vi "RichToFlatnise_StatusInfo.vi"(5 "OutputClusterType":T1, 11 "InputCluster":T2) -> (3 "OutputCluster":T1)   [LabVIEW 2021, in "basic_switch_executive_driver_client.lvlib"]
uses:
  basic_switch_executive_driver_client.lvlib
  nise_StatusInfo_Flat.ctl
  nise_StatusInfo.ctl
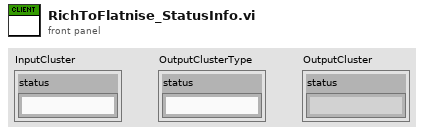
[diagram p1: front panel]
types:
  T1 = typedef "basic_switch_executive_driver_client.lvlib/nise_StatusInfo_Flat.ctl" = cluster{"status":string}
  T2 = typedef "basic_switch_executive_driver_client.lvlib/nise_StatusInfo.ctl" = cluster{"status":string}
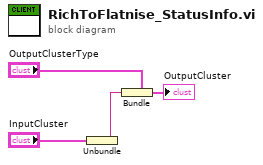
[diagram p0: block diagram]
diagram:
  n1 = Unbundle "Unbundle"("InputCluster") -> ("status"=w1:string)
  n2 = Bundle "Bundle"(cluster="OutputClusterType", "status"=w1) -> (→"OutputCluster":T1)
